vi "DSF.Memory.Buffer.Errors.vi"   [LabVIEW 2016, in "DSF.Engine.lvlib" / "DSF.Memory.Buffer.lvclass"]
uses:
  DSF.Memory.Buffer.lvclass
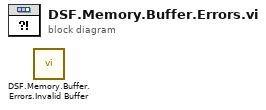
[diagram p0: block diagram]
diagram:
  n1 = call "DSF.Memory.Buffer.Errors.Invalid Buffer.vi"() -> ()  [unwired: 10 in, 2 out]
